vi "GetVersionNumberSum.vi"(8 "Error In":errorcluster) -> (0 "Error Out":errorcluster, 2 "VersionNumberSum":u64)   [LabVIEW 2020, in "16_Helper.lvclass"]
uses:
  16_Helper.lvclass
  16_Helper.lvclass/16_Helper.ctl
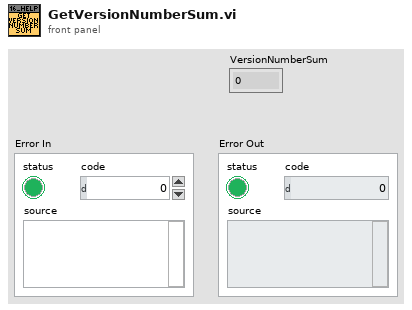
[diagram p1: front panel]
types:
  T1 = typedef "16_Helper.lvclass/ObjectAttributes.ctl" = cluster{"VersionNumberSum":u64}
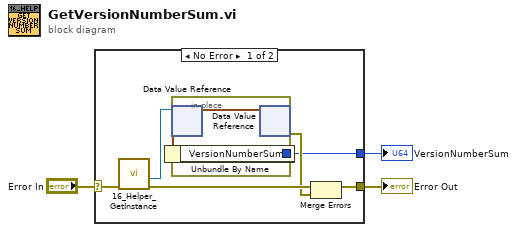
[diagram p0: block diagram]
diagram:
  n1 = case shown="No Error" "Error In" {
    selector: "Error In" -> [w9 w12]
    tunnel: [w7 w12] -> w2
    tunnel: [w5 _] -> w1
    frame No Error {
      n2 = call "16_Helper_GetInstance.vi"("error in"=w9) -> ("error out"=w8:errorcluster, "DVRRefOut"=w4:refnum<data-value>)  [unwired: 6 in, 3 out]
      n3 = in-place {
        in-place-border: [w11] -> w5
        n4 = in-place-dvr #1(w4) -> (w10:T1)  [unwired: 1 out]
        n5 = Unbundle By Name(w10) -> ("VersionNumberSum"=w11:u64)
        n6 = in-place-dvr #1(w10) -> (w6:errorcluster)  [unwired: 1 out]
      }
      n7 = Merge Errors(w8, w6) -> (w7:errorcluster)
    }
    frame Error {
    }
  }
  "Error Out" <- w2
  "VersionNumberSum" <- w1
